vi "SetLineParams.vi"(8 "error in (no error)":errorcluster, 9 "pen":T1={"Width"=1, "Style"=enum."Solid"}, 10 "color":u32(colorbox), 11 "Line in":refnum<class "Line.lvclass">) -> (0 "error out":errorcluster, 3 "Line out":refnum<class "Line.lvclass">)   [LabVIEW 2014, in "Line.lvclass"]
uses:
  Line.lvclass
  Line.lvclass/Line.ctl
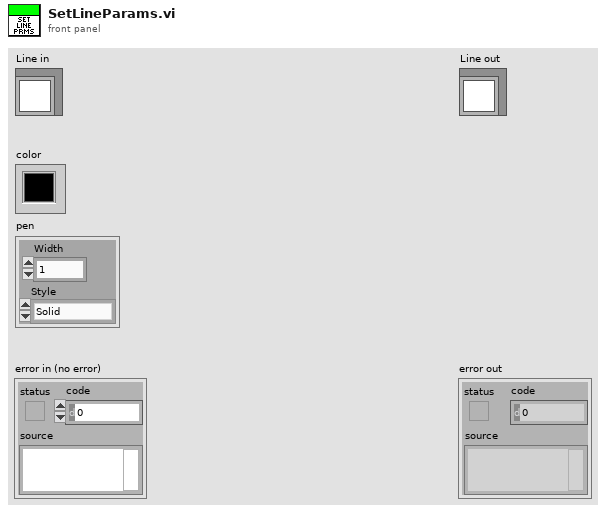
[diagram p1: front panel]
types:
  T1 = cluster{"Width":u16, "Style":enum32{"Solid", "Dash", "Dot", "DashDot", "DashDotDot"}}
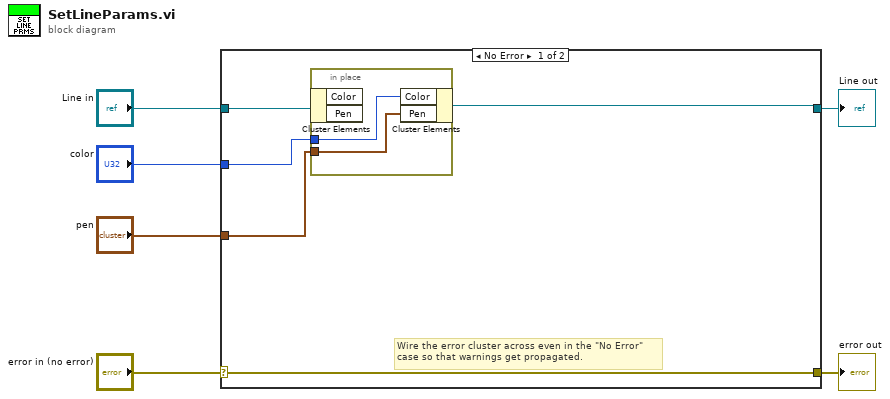
[diagram p0: block diagram]
diagram:
  n1 = case shown="No Error" "error in (no error)" {
    selector: "error in (no error)" -> [w11 w15]
    tunnel: [w11 w15] -> w5
    tunnel: [w7 w14] -> w3
    tunnel: "Line in" -> [w10 w14]
    tunnel: "pen" -> [w9 _]
    tunnel: "color" -> [w8 _]
    frame No Error {
      # "Wire the error cluster across even in the \"No Error\"\ncase so that warnings get propagated."
      n2 = in-place {
        in-place-border: w9 -> [w13]
        in-place-border: w8 -> [w12]
        n3 = in-place-cluster #1(w10) -> ()  [unwired: 2 out]
        n4 = in-place-cluster #1("Color"=w12, "Pen"=w13) -> (w7:refnum<class "Line.lvclass">)
      }
    }
    frame Error {
    }
  }
  "error out" <- w5
  "Line out" <- w3
